vi "获取设备厂家信息解析.vi"(11 "输入字符串":string) -> (3 "获取设备厂家信息":T1)   [LabVIEW 2016, in "环境动力监测库.lvlib" / "空调库.lvlib"]
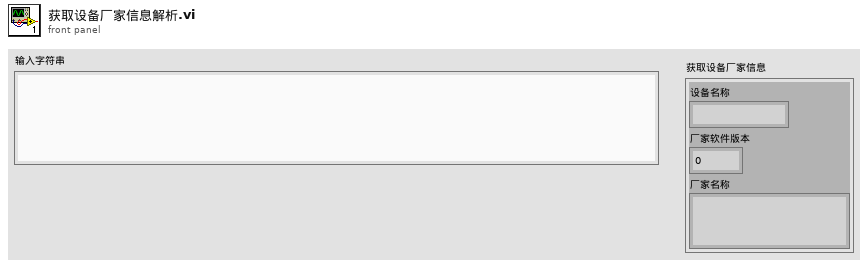
[diagram p1: front panel]
types:
  T1 = cluster{"设备名称":string, "厂家软件版本":u16, "厂家名称":string}
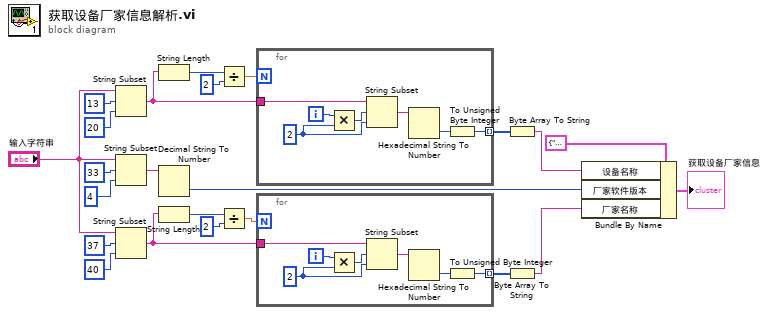
[diagram p0: block diagram]
diagram:
  n1 = String Subset(string="输入字符串", offset (0)=13 ("偏移量(0)"), length (rest)=20 ("长度（剩余）")) -> (substring=w12:string)
  n2 = String Subset(string="输入字符串", offset (0)=33 ("偏移量(0)"), length (rest)=4 ("长度（剩余）")) -> (substring=w2:string)
  n3 = String Subset(string="输入字符串", offset (0)=37 ("偏移量(0)"), length (rest)=40 ("长度（剩余）")) -> (substring=w6:string)
  n4 = String Length(string=w12) -> (length=w16:i32)
  n5 = Decimal String To Number(string=w2) -> (number=w1:i32)  [unwired: 2 in, 1 out]
  n6 = String Length(string=w6) -> (length=w7:i32)
  n7 = Divide(x=w16, y=2) -> (x/y=w14:dbl)
  n8 = Divide(x=w7, y=2) -> (x/y=w9:dbl)
  n9 = for {
    N: w14 -> [_]
    tunnel: w12 -> [w29]
    tunnel: [w24] -> w13 mode=indexing
    i -> [w28]
    w27 = 2 ("长度（剩余）")
    n10 = Multiply(x=w28, y=w27) -> (x*y=w26:i32)
    n11 = String Subset(string=w29, offset (0)=w26, length (rest)=w27) -> (substring=w30:string)
    n12 = Hexadecimal String To Number(string=w30) -> (number=w25:u32)  [unwired: 2 in, 1 out]
    n13 = To Unsigned Byte Integer(number=w25) -> (unsigned 8bit integer=w24:u8)
  }
  n14 = for {
    N: w9 -> [_]
    tunnel: w6 -> [w36]
    tunnel: [w31] -> w10 mode=indexing
    i -> [w35]
    w34 = 2 ("长度（剩余）")
    n15 = Multiply(x=w35, y=w34) -> (x*y=w33:i32)
    n16 = String Subset(string=w36, offset (0)=w33, length (rest)=w34) -> (substring=w37:string)
    n17 = Hexadecimal String To Number(string=w37) -> (number=w32:u32)  [unwired: 2 in, 1 out]
    n18 = To Unsigned Byte Integer(number=w32) -> (unsigned 8bit integer=w31:u8)
  }
  n19 = Byte Array To String(unsigned byte array=w13) -> (string=w11:string)
  n20 = Byte Array To String(unsigned byte array=w10) -> (string=w5:string)
  n21 = Bundle By Name(cluster=T1 {"设备名称"="ac\u0000\u0000\u0000\u0000\u0000\u0000\u0000\u0000", "厂家软件版本"=0, "厂家名称"="haydensuzhou\u0000\u0000\u0000\u0000\u0000\u0000\u0000\u0000"} ("获取设备厂家信息"), "设备名称"=w11, "厂家软件版本"=w1, "厂家名称"=w5) -> (→"获取设备厂家信息":T1)
